vi "INV_test results.vi"(6 "error":errorcluster, 7 "save results":bool, 8 "test pass":bool, 9 "step_type":T1, 10 "Numeric":dbl, 11 "(description) used in test":string) -> (2 "test results":T2)   [LabVIEW 2020]
uses:
  controls/INV_test results.ctl
  controls/Inverter_step_type.ctl
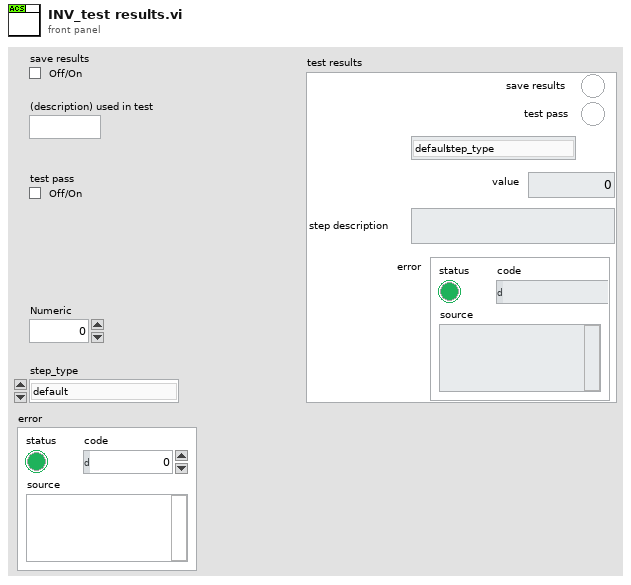
[diagram p1: front panel]
types:
  T1 = typedef "Inverter_step_type.ctl" = enum16{"default", "prompt", "init_12V_power_supply", "12V_power supply on_off", "write_PLC", "read_PLC", "DAQ_Read", "DAQ_Write", "run .bat file", "display_version", "set flow rate", "init_chroma", "set_chroma_V", "set_chroma_ramp", "wait (sec)", "end_test", "record_pass_fail"}
  T2 = typedef "INV_test results.ctl" = cluster{"test pass":bool, "step_type":T1, "value":dbl, "step description":string, "error":errorcluster, "save results":bool}
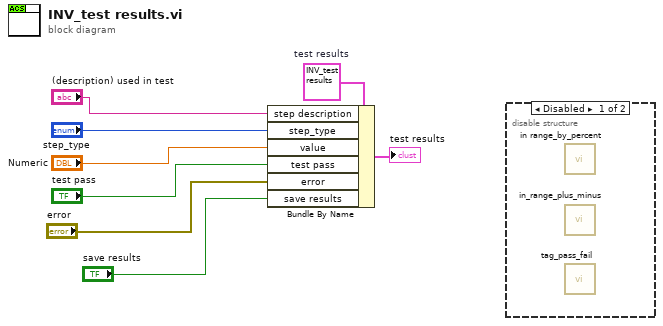
[diagram p0: block diagram]
diagram:
  w4 = T2 {"test pass"=FALSE, "step_type"=enum."prompt", "value"=0.0, "step description"="", "error"={"status"=FALSE, "code"=0, "source"=""}, "save results"=FALSE}  # test results
  n1 = Bundle By Name(cluster=w4, "step description"="(description) used in test", "step_type"="step_type", "value"="Numeric", "test pass"="test pass", "error"="error", "save results"="save results") -> (→"test results":T2)
  n2 = disable-structure shown="Disabled" {
    frame Disabled {
      n3 = call "in range_by_percent.vi"() -> ()  [unwired: 8 in, 4 out]
      n4 = call "in_range_plus_minus.vi"() -> ()  [unwired: 10 in, 2 out]
      n5 = call "tag_pass_fail.vi"() -> ()  [unwired: 11 in, 1 out]
    }
    frame Enabled {
    }
  }
